vi "boolsToString.vi"(1 "input_bool_low":bool=TRUE, 2 "input_bool_high":bool=TRUE) -> (0 "show_str_01string":string)   [LabVIEW 2011]
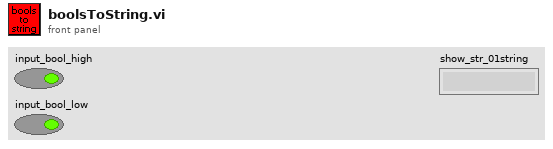
[diagram p1: front panel]
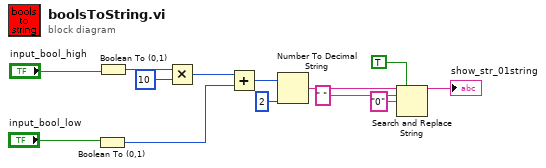
[diagram p0: block diagram]
diagram:
  n1 = Boolean To (0,1)(Boolean="input_bool_low") -> (0, 1=w8:i16)
  n2 = Boolean To (0,1)(Boolean="input_bool_high") -> (0, 1=w11:i16)
  n3 = Multiply(x=w11, y=i16 10) -> (x*y=w9:i16)
  n4 = Add(x=w9, y=w8) -> (x+y=w7:i16)
  n5 = Number To Decimal String(number=w7, width (-)=i16 2 ("宽度(-)")) -> (decimal integer string=w5:string)
  n6 = Search and Replace String(replace all?=TRUE ("替换全部？(F)"), input string=w5, search string=" " ("搜索字符串"), replace string="0" ("替换字符串(\"\")")) -> (result string=→"show_str_01string":string)  [unwired: 4 in, 3 out]
